vi "Write Reading.vi"(8 "error in (no error)":errorcluster, 10 "Reading":T1={"Reading #"=0, "Readings"=[3.9289019107818604], "Reading Name"="Splice distortion", "Type"=enum."Defect", "Alarm priority"=enum."No Alarm", "Display precision"=0}, 11 "SQLite Connection in":refnum<class "Connection.lvclass">) -> (0 "error out":errorcluster, 3 "SQLite Connection":refnum<class "Connection.lvclass">)   [LabVIEW 2017, in "Copy of Beltwatch SQLite.lvlib"]
uses:
  Beltwatch/BeltWatch 4-2-2-5/Database/Copy of Beltwatch SQLite.lvlib
  SQ Lite Cluster Action.ctl
  Beltwatch/SourceCode/BeltWatch Reading.ctl
  Beltwatch/SourceCode/BeltWatch Event type.ctl
  Beltwatch/SourceCode/BeltWatch Alarm Priority.ctl
  <vilib>/drjdpowell/SQLite Library/SQL Connection/Connection.lvclass
  <vilib>/drjdpowell/SQLite Library/SQL Statement/SQL Statement.lvclass/SQL Statement.ctl
  <vilib>/drjdpowell/SQLite Library/SQL Connection/Connection.lvclass/Connection.ctl
  <vilib>/drjdpowell/SQLite Library/SQL Statement/Bind Integer.vi
  <vilib>/drjdpowell/SQLite Library/SQL Statement/Bind Real.vi
  <vilib>/drjdpowell/SQLite Library/SQL Statement/Error Message.vi
  <vilib>/drjdpowell/SQLite Library/SQL Statement/SQL Statement.lvclass
panel:
  out "Time 2":u32
  out "size(s)":i32
  out "Numeric":i32
  out "Valtime":u32
  out "Time":u32
  out "Array":string[](array[string])
  out "Controls[]":refnum<vi>[](array[refnum])
  out "Reading SQL":string
  out "SQLite3 type":T4(ring)
  in  "ReadingsCols":T5[](array[typedef])=[{"Include"=TRUE, "Name"="Reading #", "SQLite3 type"=enum."SQLITE_INTEGER"}, {"Include"=TRUE, "Name"="Readings", "SQLite3 type"=enum."SQLITE3_TEXT"}, {"Include"=TRUE, "Name"="Reading Name", "SQLite3 type"=enum."SQLITE3_TEXT"}, {"Include"=TRUE, "Name"="TypeVal", "SQLite3 type"=enum."SQLITE_INTEGER"}, {"Include"=TRUE, "Name"="Alarm priority", "SQLite3 type"=enum."SQLITE_INTEGER"}, {"Include"=FALSE, "Name"="Display precision", "SQLite3 type"=enum."undefined type (0)"}, {"Include"=TRUE, "Name"="TypeStr", "SQLite3 type"=enum."SQLITE3_TEXT"}, {"Include"=TRUE, "Name"="AlarmPriorityStr", "SQLite3 type"=enum."SQLITE3_TEXT"}]
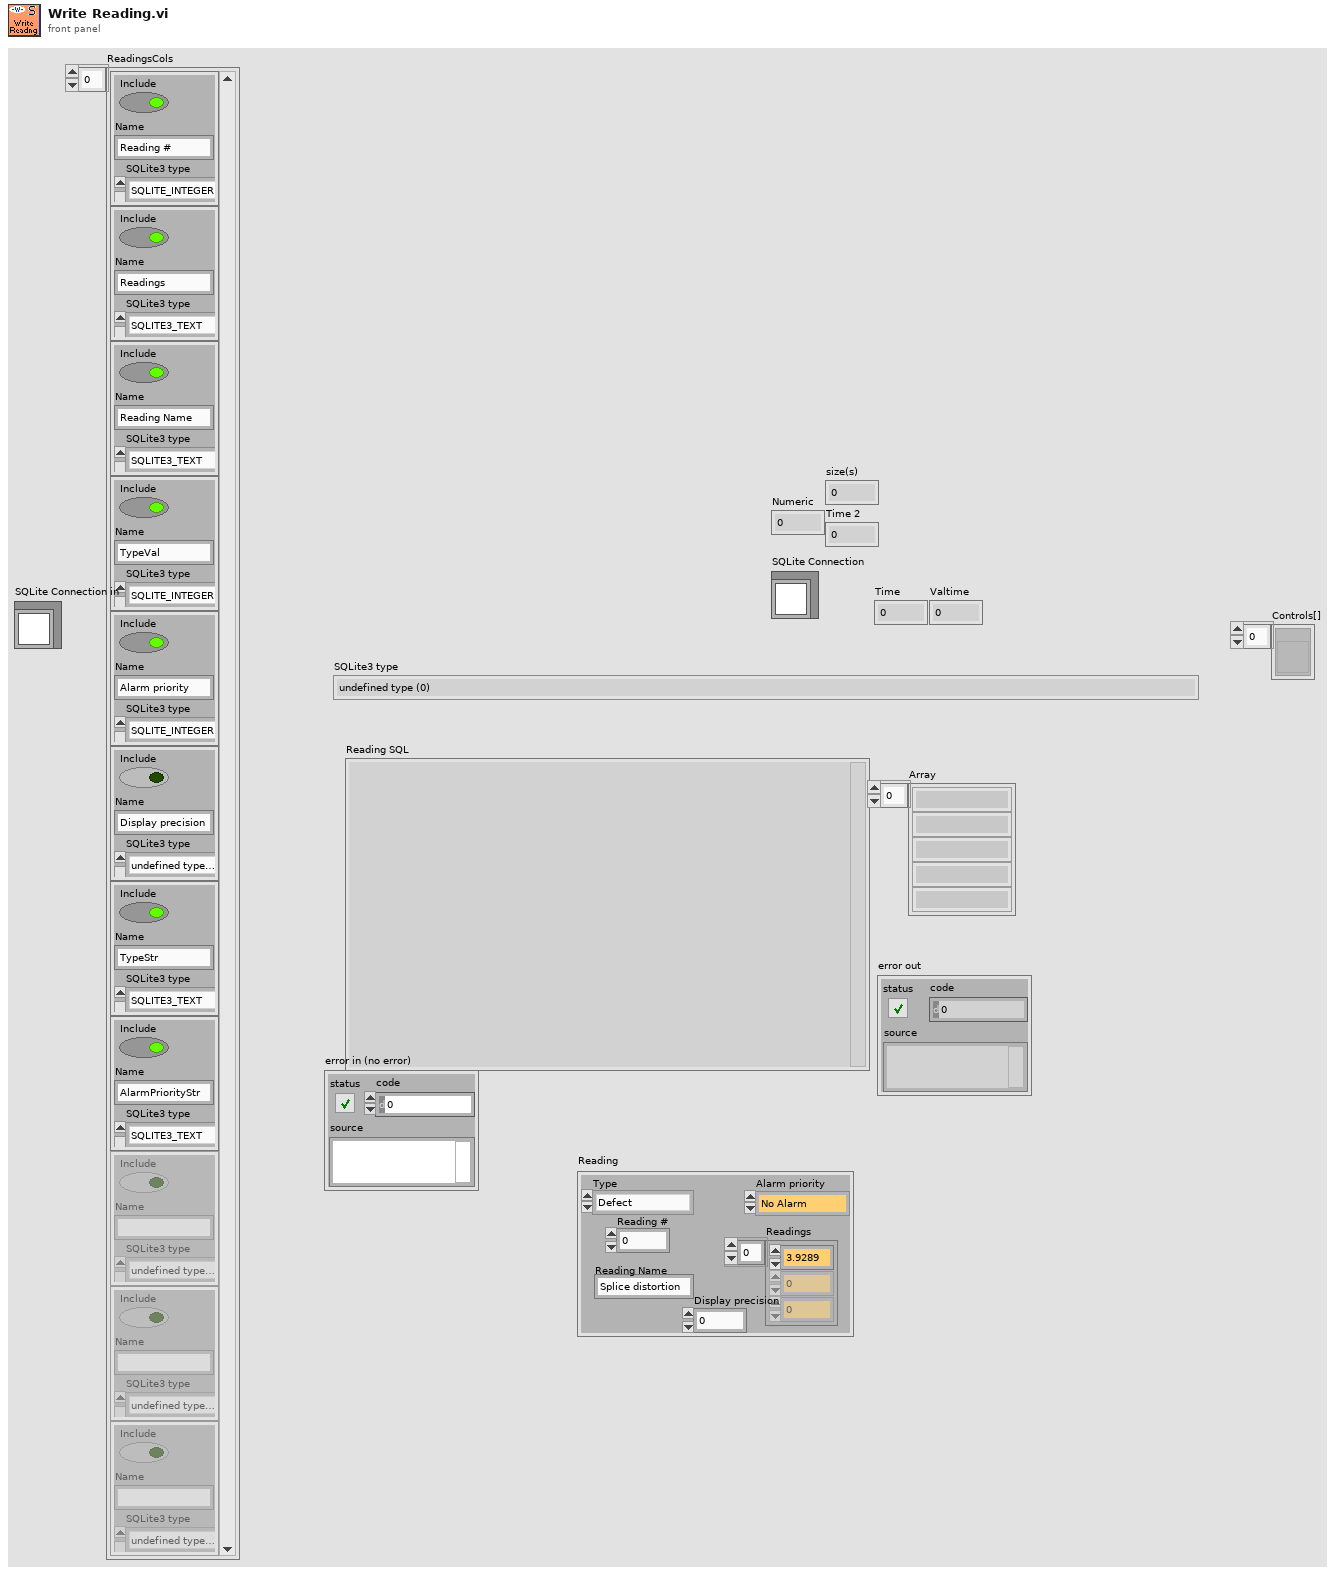
[diagram p1: front panel]
types:
  T1 = typedef "BeltWatch Reading.ctl" = cluster{"Reading #":i32, "Readings":dbl[], "Reading Name":string, "Type":T2, "Alarm priority":T3, "Display precision":i32}
  T2 = typedef "BeltWatch Event type.ctl" = enum16{"Defect", "Splice", "Break", "Rip", "Track", "Segment", "Belt", "New Splice", "Missing Splice", "None", "Free"}
  T3 = typedef "BeltWatch Alarm Priority.ctl" = enum16{"No Alarm", "High", "Medium", "Low"}
  T4 = enum32{"undefined type (0)", "SQLITE_INTEGER", "SQLITE_FLOAT", "SQLITE3_TEXT", "SQLITE_BLOB", "SQLITE_NULL", "undefined type"}
  T5 = typedef "Copy of Beltwatch SQLite.lvlib/SQ Lite Cluster Action.ctl" = cluster{"Include":bool, "Name":string, "SQLite3 type":enum32{"undefined type (0)", "SQLITE_INTEGER", "SQLITE_FLOAT", "SQLITE3_TEXT", "SQLITE_BLOB", "SQLITE_NULL", "undefined type", "FloatArray"}}
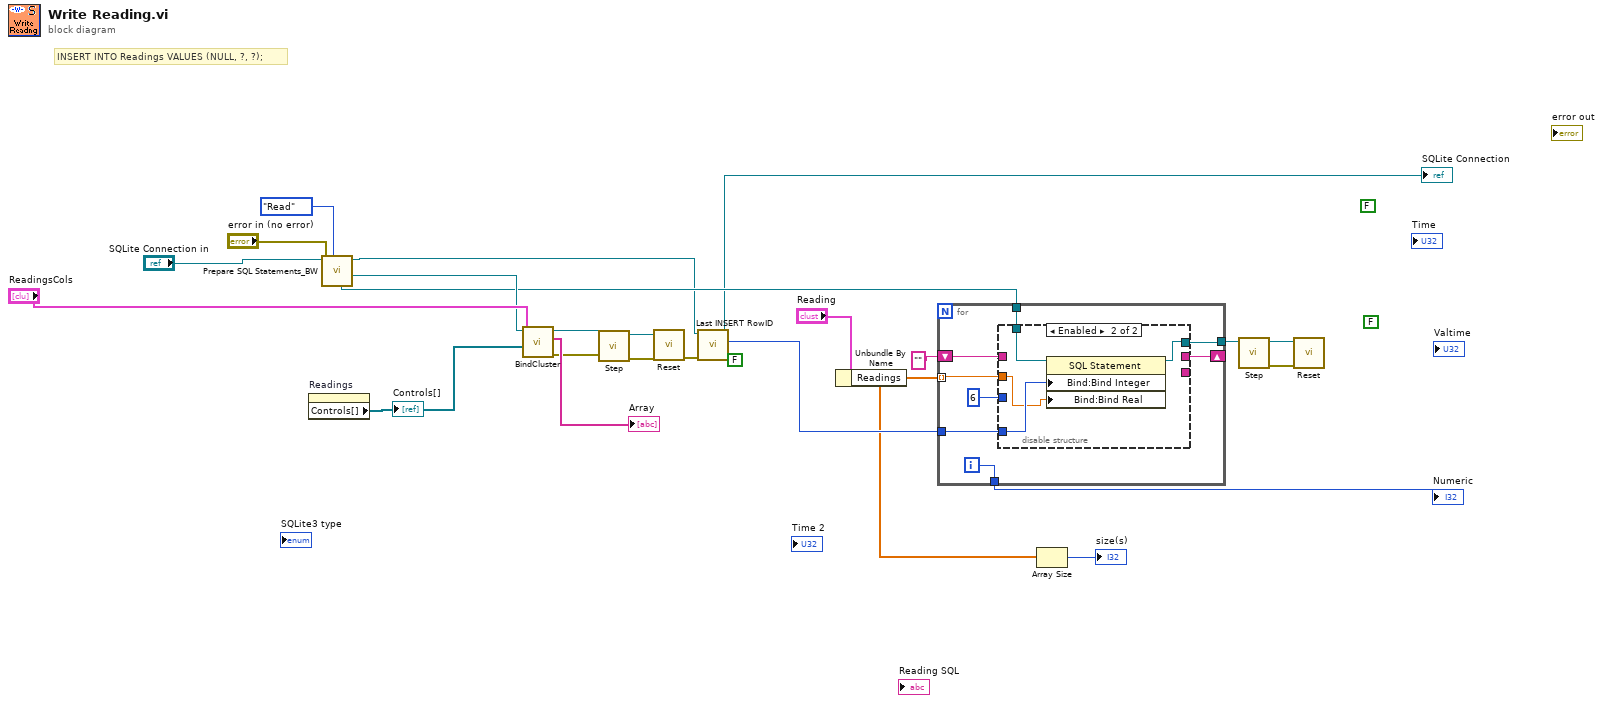
[diagram p0: block diagram]
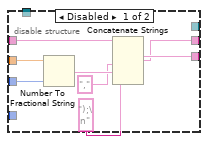
[diagram p2: hidden frame]
diagram:
  (unwired) FALSE ("UsePrevious")
  (unwired) FALSE ("UsePrevious")
  (unwired) FALSE ("UsePrevious")
  # "INSERT INTO Readings VALUES (NULL, ?, ?);"
  n1 = property on="Readings" class="Clust (strict)"() -> ("Controls[]"=w22:refnum<vi>[])  [unwired: 2 in, 2 out]
  "Controls[]" <- w22
  n2 = call "Prepare SQL Statements_BW.vi"("action"=enum16{"Init", "Read", "Finalise"}."Read", "error in (no error)"="error in (no error)", "SQLite Connection in"="SQLite Connection in") -> ("Readings"=w17:refnum<class "SQL Statement.lvclass">, "SQLite Connection out"=w5:refnum<class "Connection.lvclass">, "REadingVal"=w10:refnum<class "SQL Statement.lvclass">)  [unwired: 4 in, 2 out]
  n3 = call "BindCluster.vi"("Controls[]"=w22, "Cols"="ReadingsCols", "SQL Statement in"=w17) -> ("error out"=w12:errorcluster, "Array"=→"Array":string[], "SQL Statement out"=w16:refnum<class "SQL Statement.lvclass">)  [unwired: 5 in, 1 out]
  n4 = call <vilib>:"Step.vi"("error in (no error)"=w12, "SQL Statement in"=w16) -> ("error out"=w18:errorcluster, "SQL Statement"=w19:refnum<class "SQL Statement.lvclass">)  [unwired: 7 in, 1 out]
  n5 = call <vilib>:"Reset.vi"("error in (no error)"=w18, "SQL Statement in"=w19) -> ("error out"=w15:errorcluster)  [unwired: 8 in, 1 out]
  n6 = call <vilib>:"Last INSERT RowID.vi"("error in (no error)"=w15, "SQLite Connection in"=w5) -> ("Last INSERT RowID"=w9:i64, "SQLite Connection"=→"SQLite Connection":refnum<class "Connection.lvclass">)  [unwired: 7 in, 1 out]
  n7 = Unbundle By Name("Reading") -> ("Readings"=w3:dbl[])
  n8 = for {
    tunnel: w3 -> [w32] mode=indexing
    shift-right: [w30] -> _
    shift-left: "" -> [w29]
    tunnel: w10 -> [w28]
    tunnel: w9 -> [w27]
    tunnel: [w26] -> w7
    tunnel: [w25] -> w4
    i -> [w25]
    n9 = disable-structure shown="Enabled" {
      disable-tunnel: w32 -> [w40 w42]
      disable-tunnel: i16 6 ("precision (6)") -> [w39 _]
      disable-tunnel: _ -> [w38 _]
      disable-tunnel: [w34 _] -> w30
      disable-tunnel: w29 -> [w33 _]
      disable-tunnel: w28 -> [_ w44]
      disable-tunnel: w27 -> [_ w43]
      disable-tunnel: [_ w41] -> w26
      frame Disabled {
        n10 = Number To Fractional String(number=w40, precision (6)=w39) -> (F-format string=w37:string)  [unwired: 2 in]
        n11 = Concatenate Strings(w33, w38, "," ("string"), w37, ");\n" ("string")) -> (w34:string)  [unwired: 1 in]
      }
      frame Enabled {
        n12 = property class="SQL Statement"(reference=w44, "Bind:Bind Integer"=w43, "Bind:Bind Real"=w42) -> (reference out=w41:refnum<class "SQL Statement.lvclass">)  [unwired: 1 in, 1 out]
      }
    }
  }
  "Numeric" <- w4
  n13 = Array Size(array=w3) -> (size(s)=→"size(s)":i32)
  n14 = call <vilib>:"Step.vi"("SQL Statement in"=w7) -> ("error out"=w8:errorcluster, "SQL Statement"=w6:refnum<class "SQL Statement.lvclass">)  [unwired: 8 in, 1 out]
  n15 = call <vilib>:"Reset.vi"("error in (no error)"=w8, "SQL Statement in"=w6) -> ()  [unwired: 8 in, 2 out]
